vi "pl1000OpenUnitProgress.vi"(8 "error in (no error)":errorcluster) -> (0 "error out":errorcluster, 1 "complete":bool, 2 "progress":i32, 3 "pl1000 handle out":i16)   [LabVIEW 2016, in "pl1000.lvlib"]
uses:
  pl1000.lvlib
  pl1000.dll
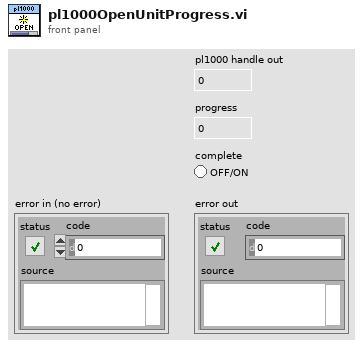
[diagram p1: front panel]
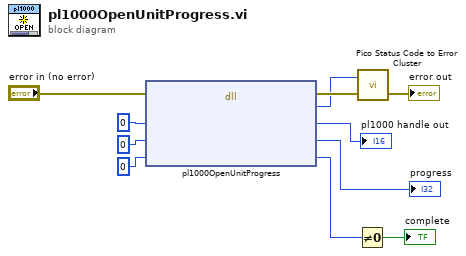
[diagram p0: block diagram]
diagram:
  n1 = dll-call lib="pl1000.dll" fn="pl1000OpenUnitProgress"(error in="error in (no error)", "handle"=i16 0, "progress"=0, "complete"=0) -> (error out=w9:errorcluster, "status"=w8:u32, "handle"=→"pl1000 handle out":i16, "progress"=→"progress":i32, "complete"=w2:i32)  [unwired: 2 in, 1 out]
  n2 = Not Equal To 0?(x=w2) -> (x != 0?=→"complete":bool)
  n3 = call "Pico Status Code to Error Cluster.vi"("error in"=w9, "PICO_STATUS"=w8) -> ("error out"=→"error out":errorcluster)  [unwired: 1 in]
